vi "selection_is_target.vi"(8 "error in":errorcluster, 11 "vs_tree_control in":refnum<class "vs_tree_control.lvclass">) -> (0 "error out":errorcluster, 2 "is target?":bool, 3 "vs_tree_control out":refnum<class "vs_tree_control.lvclass">)   [LabVIEW 2020, in "vs_tree_control.lvclass"]
uses:
  vs_tree_control.lvclass
  NationalInstruments.VeriStand.SystemDefinitionAPI
panel:
  out "error out 2":errorcluster
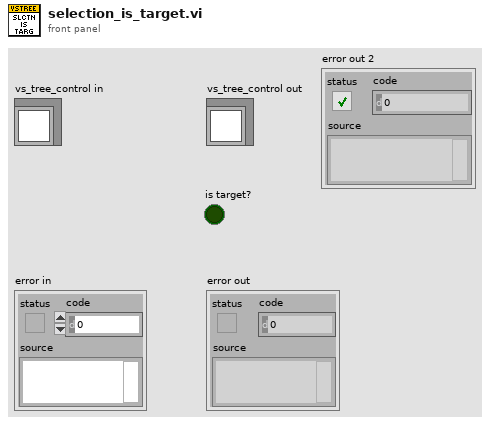
[diagram p1: front panel]
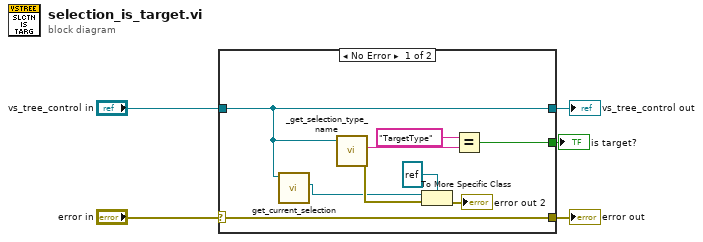
[diagram p0: block diagram]
diagram:
  n1 = case shown="No Error" "error in" {
    selector: "error in" -> [w14 w16]
    tunnel: [w14 w16] -> w4
    tunnel: [w9 w15] -> w2
    tunnel: "vs_tree_control in" -> [w9 w15]
    tunnel: [w11 _] -> w1
    frame No Error {
      n2 = call "get_current_selection.vi"("vs_tree_control in"=w9) -> ("Selection Reference"=w8:refnum<k24>)  [unwired: 7 in, 3 out]
      n3 = call "_get_selection_type_name.vi"("vs_tree_control in"=w9) -> ("error out"=w10:errorcluster, "TypeName"=w13:string)  [unwired: 8 in, 1 out]
      n4 = To More Specific Class(target class=refnum<k24> refnum, reference=w8, error in=w10) -> (error out=→"error out 2":errorcluster)  [unwired: 1 out]
      n5 = Equal?(x="TargetType", y=w13) -> (x = y?=w11:bool)
    }
    frame Error {
    }
  }
  "error out" <- w4
  "vs_tree_control out" <- w2
  "is target?" <- w1
